vi "SaveData No Objects.vi"(8 "error in (no error)":errorcluster, 9 "Comments":string="Comment Thread", 10 "File Name":path, 11 "Synapse CCD in":T1={"JYCCDLib.IJYCCDReqd"=refnum, "JYMONOLib.IJYMonoReqd"=refnum, "Integration time"=0.01, "ADC"=0, "GAIN"=0, "areas :"=[[1, 1, 1, 1024, 256, 1, 256]], "Most Recent Data Object"=refnum, "Mono Properties"={"Grating"=0, "Center Wavelength"=0.0, "Entrance Slit"=0.0, "Exit Slit"=0.0}, "Coverage"={"Max"=0.0, "Min"=0.0}, "Multi-Acquisitions"={"Dark Subtract?"=FALSE, "Averaging?"=FALSE, "Cosmic Ray Removal?"=FALSE, "# to Average"=0, "Time Between Acq."=0, "Acquisitions Control Array"=[TRUE], "Raw Data"=[], "Processed Data"=[], "Array of Wavelengths"=[]}, "Channel Names"=["Wavelength", "Signal"], "Channel Units"=["nm", "counts"]} {"ADC" items=["   20 kHz", "1 MHz", "1 MHz Ultra"]; "GAIN" items=["High Light", "Best Dynamic", "High Sensitivity"]; "Mono Properties"."Grating" items=["1200 lines/mm - 500 nm Blaze", "1200 lines/mm - 750 nm Blaze", "600 lines/mm - 1000 nm Blaze"]}) -> (0 "error out":errorcluster, 3 "Synapse CCD out":T1={"JYCCDLib.IJYCCDReqd"=refnum, "JYMONOLib.IJYMonoReqd"=refnum, "Integration time"=0.01, "ADC"=0, "GAIN"=0, "areas :"=[[1, 1, 1, 1024, 256, 1, 256]], "Most Recent Data Object"=refnum, "Mono Properties"={"Grating"=0, "Center Wavelength"=0.0, "Entrance Slit"=0.0, "Exit Slit"=0.0}, "Coverage"={"Max"=0.0, "Min"=0.0}, "Multi-Acquisitions"={"Dark Subtract?"=FALSE, "Averaging?"=FALSE, "Cosmic Ray Removal?"=FALSE, "# to Average"=0, "Time Between Acq."=0, "Acquisitions Control Array"=[TRUE], "Raw Data"=[], "Processed Data"=[], "Array of Wavelengths"=[]}, "Channel Names"=["Wavelength", "Signal"], "Channel Units"=["nm", "counts"]} {"ADC" items=["   20 kHz", "1 MHz", "1 MHz Ultra"]; "GAIN" items=["High Light", "Best Dynamic", "High Sensitivity"]; "Mono Properties"."Grating" items=["1200 lines/mm - 500 nm Blaze", "1200 lines/mm - 750 nm Blaze", "600 lines/mm - 1000 nm Blaze"]})   [LabVIEW 2009]
doc: "Packages Processed and Raw Data for Export to Excel.vi"
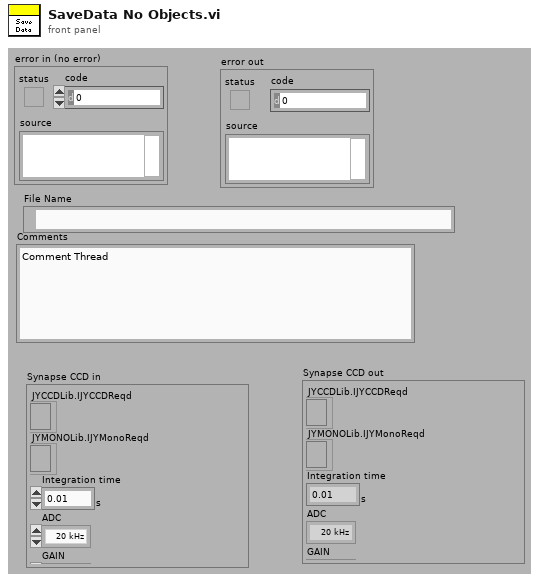
[diagram p1: front panel]
types:
  T1 = cluster{"JYCCDLib.IJYCCDReqd":refnum<k7>, "JYMONOLib.IJYMonoReqd":refnum<k7>, "Integration time":dbl[unit], "ADC":u16, "GAIN":u16, "areas :":i32[][], "Most Recent Data Object":refnum<k7>, "Mono Properties":cluster{"Grating":u16, "Center Wavelength":dbl[unit], "Entrance Slit":dbl[unit], "Exit Slit":dbl[unit]}, "Coverage":cluster{"Max":dbl[unit], "Min":dbl[unit]}, "Multi-Acquisitions":cluster{"Dark Subtract?":bool, "Averaging?":bool, "Cosmic Ray Removal?":bool, "# to Average":u32, "Time Between Acq.":u32, "Acquisitions Control Array":bool[], "Raw Data":i32[][], "Processed Data":dbl[], "Array of Wavelengths":dbl[]}, "Channel Names":string[], "Channel Units":string[]}
  T2 = typedef "Readable.lvclass/Channel Names.ctl" = string[]
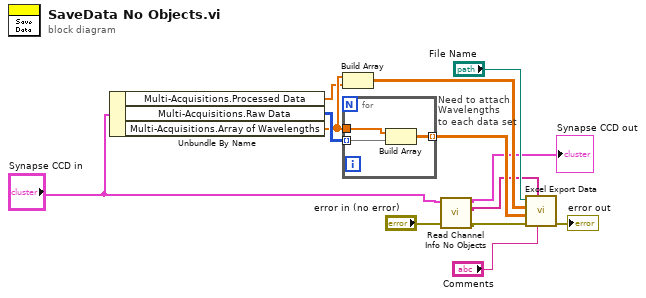
[diagram p0: block diagram]
diagram:
  n1 = Unbundle By Name("Synapse CCD in") -> ("Multi-Acquisitions.Processed Data"=w8:dbl[], "Multi-Acquisitions.Raw Data"=w11:i32[][], "Multi-Acquisitions.Array of Wavelengths"=w9:dbl[])
  n2 = Build Array(w9, w8) -> (w6:dbl[][])
  n3 = for "Need to attach Wavelengths\nto each data set" {
    tunnel: w11 -> [w15] mode=indexing
    tunnel: w9 -> [w16]
    tunnel: [w14] -> w10 mode=indexing
    n4 = Build Array(w16, w15) -> (w14:dbl[][])
  }
  n5 = call "Read Channel Info No Objects.vi"("error in (no error)"="error in (no error)", "Synapse CCD in"="Synapse CCD in") -> ("error out"=w4:errorcluster, "Channel Names"=w3:T2, "Synapse CCD out"=→"Synapse CCD out":T1)  [unwired: 5 in, 2 out]
  n6 = call "Excel Export Data.vi"("Comments"="Comments", "Channel Names"=w3, "error in (no error)"=w4, "Raw Data"=w10, "Processed Data"=w6, "File Name"="File Name") -> ("error out"=→"error out":errorcluster)  [unwired: 5 in]
